vi "Get SpinEcho Params.vi"(11 "Spin Echo Parameters":T1={"Path to Spin Echo Burner"=path "C:/Users/Loncar/Desktop/ESR VIs - Srujan/Sam Kim/PB/SpinEchoBurn.exe", "Window 1 time (s)"=3e-06, "Window 1 active channels"=[FALSE, FALSE, FALSE, TRUE], "Window 10 time (s)"=3e-06, "Window 10 active channels"=[FALSE, FALSE, FALSE, TRUE], "# samples"=0, "Window 2 time (s)"=5e-06, "Window 2 active channels"=[], "Window 4 min time (s) "=0.0, "Window 4 active channels"=[FALSE], "Window 8 time (s)"=7.5e-07, "Window 8 active channels"=[FALSE, FALSE, FALSE, TRUE], "Window 9 time (s)"=2e-07, "Window 9 active channels "=[FALSE, FALSE, TRUE, TRUE], "# time axis points"=0, "Window 11 time (s)"=2e-07, "Window 11 active channels"=[FALSE, FALSE, TRUE, TRUE], "Window 12 time (s)"=1e-07, "Window 12 active channels"=[], "Window 4 max time (s)"=0.0, "Window 3 time (s)"=5e-06, "Window 5 time (s)"=5e-06, "Window 3 active channels"=[TRUE, FALSE, FALSE, FALSE], "Window 5 active channels"=[TRUE, FALSE, FALSE, FALSE], "Window 7 time (s)"=5e-06, "Window 7 active channels"=[TRUE, FALSE, FALSE, FALSE]}) -> (0 "max time":dbl, 1 "min time":dbl, 2 "# time points":i32, 3 "# samples":i32, 4 "Window Params Args":string)   [LabVIEW 2012]
uses:
  Spin Echo Window Parameters.ctl
panel:
  # "Green AOM"
  # "Initialization"
  # "All off"
  # "Wait"
  # "MW"
  # "MW pulse 1"
  # "All off"
  # "Free precession 1"
  # "max: ~350"
  # "MW pulse 2"
  # "MW"
  # "Free precession 2: Window 6"
  # "MW"
  # "MW pulse 1"
  # "Green AOM"
  # "Wait"
  # "Green AOM,\ncounter sample clk"
  # "Readout"
  # "Green AOM"
  # "Repump"
  # "Green AOM,\ncounter sample clk"
  # "Reference"
  # "Wait (nominal)"
  # "All off"
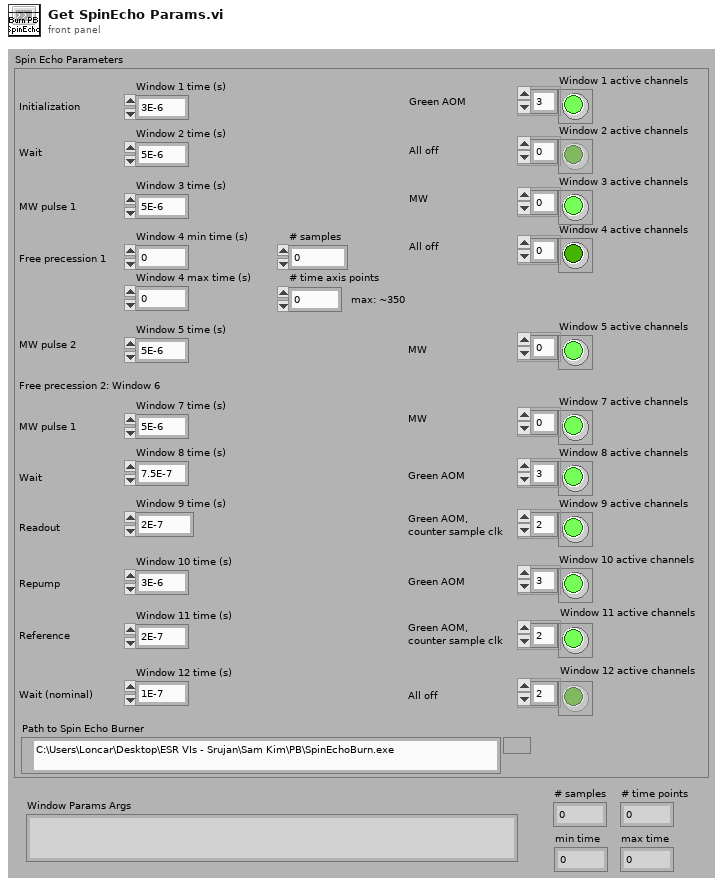
[diagram p1: front panel]
types:
  T1 = typedef "Spin Echo Window Parameters.ctl" = cluster{"Path to Spin Echo Burner":path, "Window 1 time (s)":dbl, "Window 1 active channels":bool[], "Window 10 time (s)":dbl, "Window 10 active channels":bool[], "# samples":i32, "Window 2 time (s)":dbl, "Window 2 active channels":bool[], "Window 4 min time (s) ":dbl, "Window 4 active channels":bool[], "Window 8 time (s)":dbl, "Window 8 active channels":bool[], "Window 9 time (s)":dbl, "Window 9 active channels ":bool[], "# time axis points":i32, "Window 11 time (s)":dbl, "Window 11 active channels":bool[], "Window 12 time (s)":dbl, "Window 12 active channels":bool[], "Window 4 max time (s)":dbl, "Window 3 time (s)":dbl, "Window 5 time (s)":dbl, "Window 3 active channels":bool[], "Window 5 active channels":bool[], "Window 7 time (s)":dbl, "Window 7 active channels":bool[]}
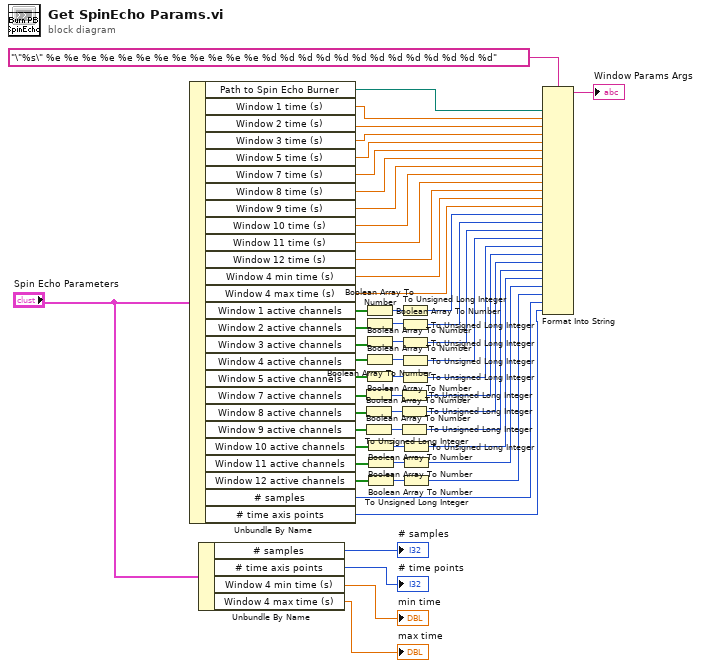
[diagram p0: block diagram]
diagram:
  n1 = Unbundle By Name("Spin Echo Parameters") -> ("Path to Spin Echo Burner"=w46:path, "Window 1 time (s)"=w50:dbl, "Window 2 time (s)"=w49:dbl, "Window 3 time (s)"=w48:dbl, "Window 5 time (s)"=w47:dbl, "Window 7 time (s)"=w45:dbl, "Window 8 time (s)"=w44:dbl, "Window 9 time (s)"=w43:dbl, "Window 10 time (s)"=w42:dbl, "Window 11 time (s)"=w41:dbl, "Window 12 time (s)"=w25:dbl, "Window 4 min time (s)"=w24:dbl, "Window 4 max time (s)"=w23:dbl, "Window 1 active channels"=w40:bool[], "Window 2 active channels"=w35:bool[], "Window 3 active channels"=w34:bool[], "Window 4 active channels"=w33:bool[], "Window 5 active channels"=w32:bool[], "Window 7 active channels"=w22:bool[], "Window 8 active channels"=w21:bool[], "Window 9 active channels"=w20:bool[], "Window 10 active channels"=w16:bool[], "Window 11 active channels"=w15:bool[], "Window 12 active channels"=w14:bool[], "# samples"=w7:i32, "# time axis points"=w6:i32)
  n2 = Unbundle By Name("Spin Echo Parameters") -> ("# samples"=→"# samples":i32, "# time axis points"=→"# time points":i32, "Window 4 min time (s)"=→"min time":dbl, "Window 4 max time (s)"=→"max time":dbl)
  n3 = Boolean Array To Number(Boolean array=w22) -> (number=w54:u32)
  n4 = Boolean Array To Number(Boolean array=w21) -> (number=w53:u32)
  n5 = Boolean Array To Number(Boolean array=w20) -> (number=w52:u32)
  n6 = Boolean Array To Number(Boolean array=w40) -> (number=w51:u32)
  n7 = Boolean Array To Number(Boolean array=w35) -> (number=w39:u32)
  n8 = Boolean Array To Number(Boolean array=w34) -> (number=w38:u32)
  n9 = Boolean Array To Number(Boolean array=w33) -> (number=w37:u32)
  n10 = Boolean Array To Number(Boolean array=w32) -> (number=w36:u32)
  n11 = Boolean Array To Number(Boolean array=w16) -> (number=w19:u32)
  n12 = Boolean Array To Number(Boolean array=w15) -> (number=w18:u32)
  n13 = Boolean Array To Number(Boolean array=w14) -> (number=w17:u32)
  n14 = To Unsigned Long Integer(number=w54) -> (unsigned 32bit integer=w13:u32)
  n15 = To Unsigned Long Integer(number=w53) -> (unsigned 32bit integer=w12:u32)
  n16 = To Unsigned Long Integer(number=w52) -> (unsigned 32bit integer=w8:u32)
  n17 = To Unsigned Long Integer(number=w51) -> (unsigned 32bit integer=w31:u32)
  n18 = To Unsigned Long Integer(number=w39) -> (unsigned 32bit integer=w30:u32)
  n19 = To Unsigned Long Integer(number=w38) -> (unsigned 32bit integer=w29:u32)
  n20 = To Unsigned Long Integer(number=w37) -> (unsigned 32bit integer=w28:u32)
  n21 = To Unsigned Long Integer(number=w36) -> (unsigned 32bit integer=w27:u32)
  n22 = To Unsigned Long Integer(number=w19) -> (unsigned 32bit integer=w9:u32)
  n23 = To Unsigned Long Integer(number=w18) -> (unsigned 32bit integer=w10:u32)
  n24 = To Unsigned Long Integer(number=w17) -> (unsigned 32bit integer=w11:u32)
  n25 = Format Into String(format string="\"%s\" %e %e %e %e %e %e %e %e %e %e %e %e %d %d %d %d %d %d %d %d %d %d %d %d %d", w46, w50, w49, w48, w47, w45, w44, w43, w42, w41, w25, w24, w23, w31, w30, w29, w28, w27, w13, w12, w8, w9, w10, w11, w7, w6) -> (resulting string=→"Window Params Args":string)  [unwired: 2 in, 1 out]
